vi "autoMaintainCurrentInstructions.vi"(6 "error in (no error)":errorcluster, 7 "MotionProfile acceleration":dbl[](array[numeric]), 8 "MotionProfile speed":dbl[](array[numeric]), 9 "running commands":string[][](array[string])) -> (0 "error out":errorcluster, 3 "running commands out":string[][](array[string]))   [LabVIEW 2012]
uses:
  <vilib>/addons/control/pid/pid.llb/PID (DBL).vi
  <vilib>/addons/control/pid/NI_PID_pid.lvlib
panel:
  in  "gyro PID":T1={"proportional gain (Kc)"=0.03, "integral time (Ti, min)"=0.01, "derivative time (Td, min)"=0.0} {"derivative time (Td, min)" format="%.3f"; "integral time (Ti, min)" format="%.3f"; "proportional gain (Kc)" format="%.3f"}
  in  "BasicDriveOffset 2":dbl=1.07
  in  "visionDrive output range":cluster{"output high":dbl, "output low":dbl}={"output high"=0.3, "output low"=-0.3} {"output low" format="%.2f"; "output high" format="%.2f"}
  in  "visionDrive PID":T1={"proportional gain (Kc)"=-2.5, "integral time (Ti, min)"=0.0, "derivative time (Td, min)"=0.0} {"derivative time (Td, min)" format="%.3f"; "integral time (Ti, min)" format="%.3f"; "proportional gain (Kc)" format="%.3f"}
  in  "manualDrivePID":T1={"proportional gain (Kc)"=1.0, "integral time (Ti, min)"=0.01, "derivative time (Td, min)"=0.0} {"derivative time (Td, min)" format="%.3f"; "integral time (Ti, min)" format="%.3f"; "proportional gain (Kc)" format="%.3f"}
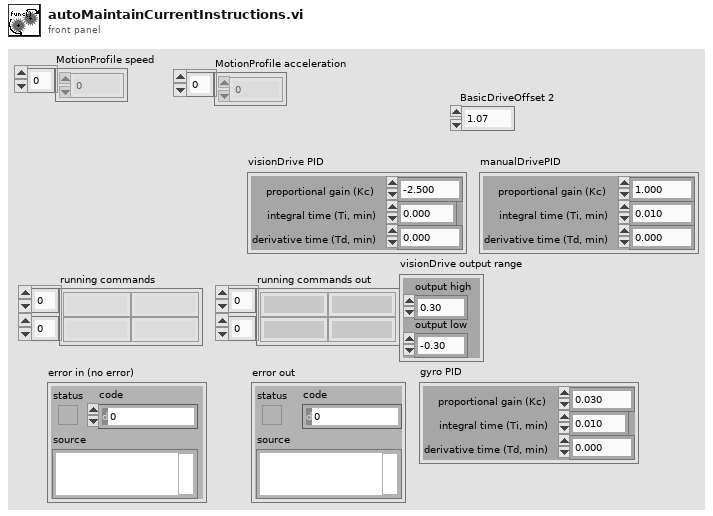
[diagram p1: front panel]
types:
  T1 = cluster{"proportional gain (Kc)":dbl, "integral time (Ti, min)":dbl, "derivative time (Td, min)":dbl}
  T2 = typedef "WPI_GyroDevRef.ctl" = cluster{"DevStatus":errorcluster, "Analog Module":T3, "Analog Channel":T4, "Offset":dbl, "Gain (VoltsPerDegree/Second)":dbl}
  T3 = typedef "FPGA_TypedefAnalogModule.ctl" = enum16{"Analog Module 1", "Analog Module 2"}
  T4 = typedef "FPGA_AIChannel.ctl" = enum8{"AI 1", "AI 2", "AI 3", "AI 4", "AI 5", "AI 6", "AI 7", "AI 8", "Invalid"}
  T5 = typedef "WPI_EncoderDevRef.ctl" = cluster{"DevStatus":errorcluster, "EncoderIndex":T6, "CounterIndex":T7, "DistancePerCount":dbl, "Decoding Type":T8}
  T6 = typedef "FPGA_EncoderIdx.ctl" = enum8{"Enc 0", "Enc 1", "Enc 2", "Enc 3", "Invalid"}
  T7 = typedef "FPGA_CounterCtrSystemIndex.ctl" = enum8{"Ctr 0", "Ctr 1", "Ctr 2", "Ctr 3", "Ctr 4", "Ctr 5", "Ctr 6", "Ctr 7", "Invalid"}
  T8 = typedef "WPI_EncoderType.ctl" = enum16{"1x", "2x", "4x"}
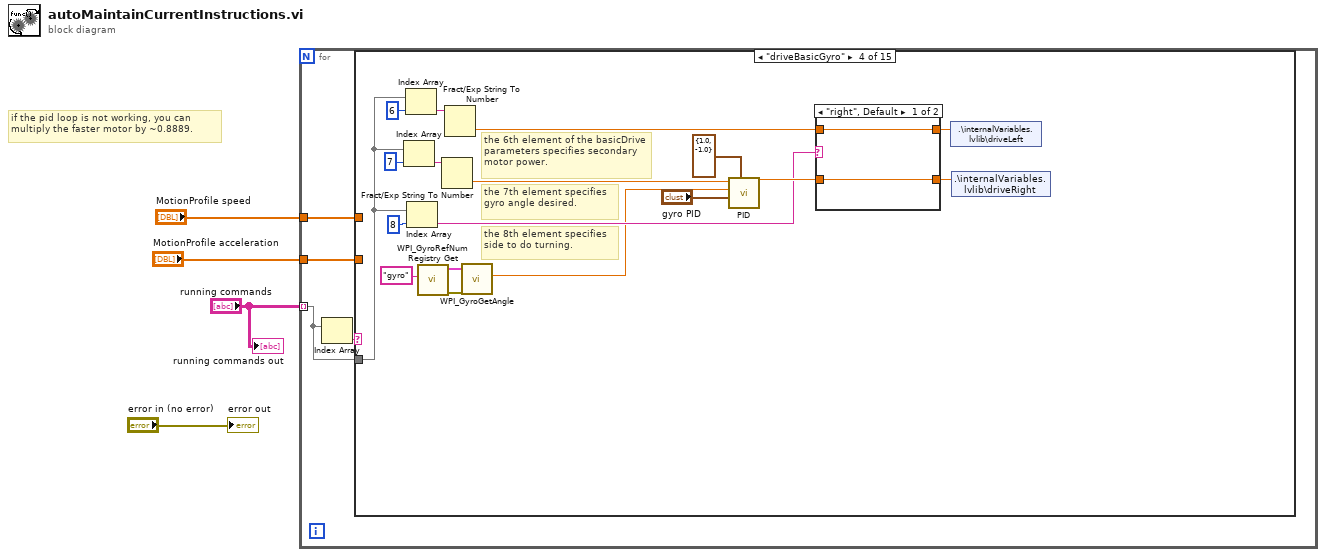
[diagram p0: block diagram]
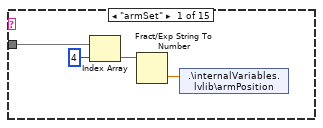
[diagram p2: hidden frame]
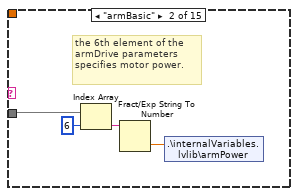
[diagram p3: hidden frame]
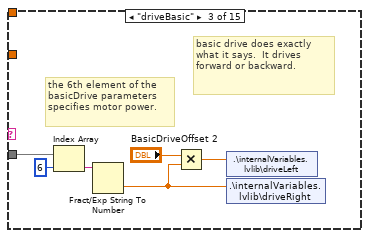
[diagram p4: hidden frame]
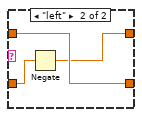
[diagram p5: hidden frame]
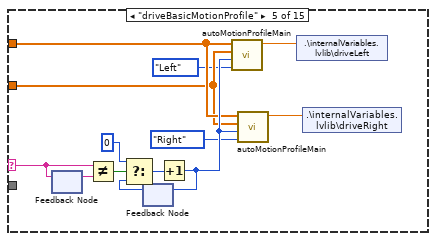
[diagram p6: hidden frame]
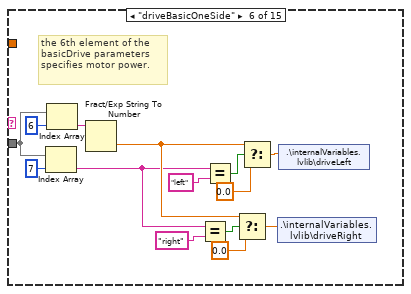
[diagram p7: hidden frame]
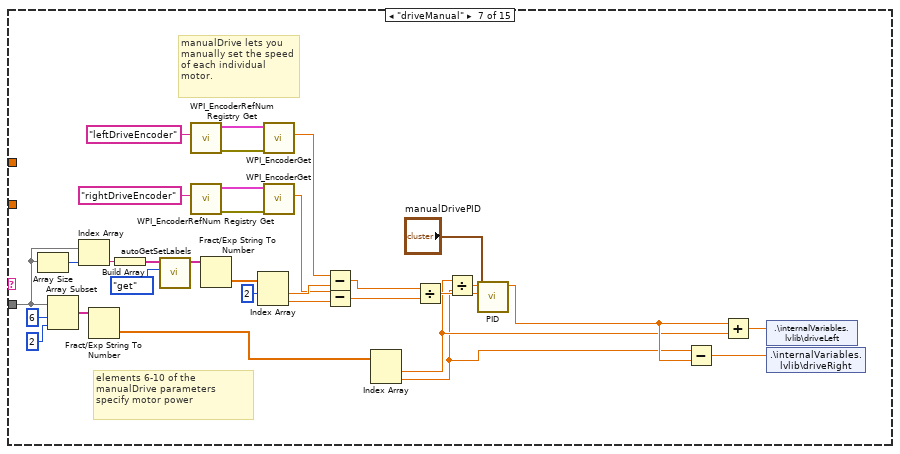
[diagram p8: hidden frame]
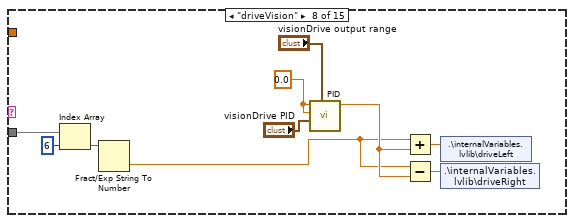
[diagram p9: hidden frame]
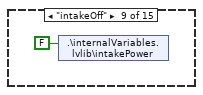
[diagram p10: hidden frame]
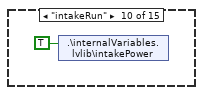
[diagram p11: hidden frame]
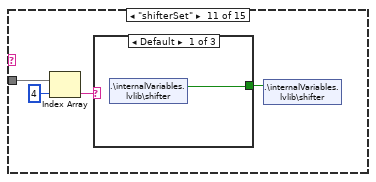
[diagram p12: hidden frame]
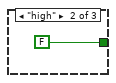
[diagram p13: hidden frame]
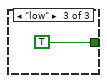
[diagram p14: hidden frame]
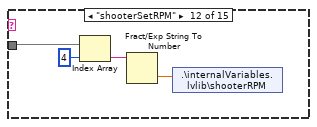
[diagram p15: hidden frame]
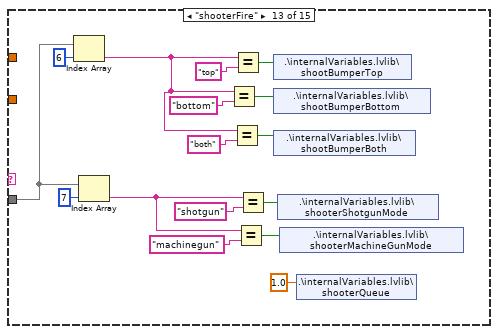
[diagram p16: hidden frame]
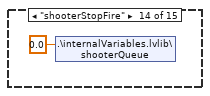
[diagram p17: hidden frame]
diagram:
  # "if the pid loop is not working, you can multiply the faster motor by ~0.8889."
  n1 = for {
    tunnel: "running commands" -> [w7] mode=indexing
    tunnel: "MotionProfile speed" -> [w6]
    tunnel: "MotionProfile acceleration" -> [w5]
    n2 = Index Array(array=w7) -> (element=w8:string)  [unwired: 1 in]
    n3 = case shown="\"driveBasicGyro\"" w8 {
      selector: w8 -> [_ _ _ _ w58 _ _ _ _ _ _ _ _ _ _]
      tunnel: w7 -> [w10 w13 w18 w34 _ w69 w96 w107 _ _ w120 w126 w134 _ _]
      tunnel: w6 -> [_ _ _ _ w49 _ _ _ _ _ _ _ _ _ _]
      tunnel: w5 -> [_ _ _ _ w48 _ _ _ _ _ _ _ _ _ _]
      frame "armSet" {
        n4 = Index Array(array=w10, index=4) -> (element=w12:string)
        n5 = Fract/Exp String To Number(string=w12) -> (number=w9:dbl)  [unwired: 3 in, 1 out]
        n6 = shared-variable ".\\internalVariables.lvlib\\armPosition"(w9) -> ()  [unwired: 1 in, 1 out]
      }
      frame "armBasic" {
        # "the 6th element of the armDrive parameters specifies motor power."
        n7 = Index Array(array=w13, index=6) -> (element=w15:string)
        n8 = Fract/Exp String To Number(string=w15) -> (number=w14:dbl)  [unwired: 3 in, 1 out]
        n9 = shared-variable ".\\internalVariables.lvlib\\armPower"(w14) -> ()  [unwired: 1 in, 1 out]
      }
      frame "driveBasic" {
        # "basic drive does exactly what it says.  It drives forward or backward."
        # "the 6th element of the basicDrive parameters specifies motor power."
        n10 = Index Array(array=w18, index=6) -> (element=w21:string)
        n11 = Fract/Exp String To Number(string=w21) -> (number=w17:dbl)  [unwired: 3 in, 1 out]
        n12 = Multiply(x="BasicDriveOffset 2", y=w17) -> (x*y=w20:dbl)
        n13 = shared-variable ".\\internalVariables.lvlib\\driveLeft"(w20) -> ()  [unwired: 1 in, 1 out]
        n14 = shared-variable ".\\internalVariables.lvlib\\driveRight"(w17) -> ()  [unwired: 1 in, 1 out]
      }
      frame "driveBasicGyro" {
        # "the 8th element specifies side to do turning."
        # "the 7th element specifies gyro angle desired."
        # "the 6th element of the basicDrive parameters specifies secondary motor power."
        n15 = Index Array(array=w34, index=7) -> (element=w35:string)
        n16 = Index Array(array=w34, index=6) -> (element=w39:string)
        n17 = Index Array(array=w34, index=8) -> (element=w28:string)
        n18 = call <vilib>:"WPI_GyroRefNum Registry Get.vi"("refnum name"="gyro") -> ("error out"=w26:errorcluster, "GyroDevRef"=w25:T2)  [unwired: 9 in]
        n19 = Fract/Exp String To Number(string=w35) -> (number=w27:dbl)  [unwired: 3 in, 1 out]
        n20 = Fract/Exp String To Number(string=w39) -> (number=w31:dbl)  [unwired: 3 in, 1 out]
        n21 = call <vilib>:"WPI_GyroGetAngle.vi"("error in (no error)"=w26, "GyroDevRef"=w25) -> ("Angle"=w24:dbl)  [unwired: 6 in, 3 out]
        n22 = call-poly <vilib>:"PID.vi"("output range"=cluster{"output high":dbl, "output low":dbl} {"output high"=1.0, "output low"=-1.0}, "PID gains"="gyro PID", "process variable"=w24, "setpoint"=w27) -> ("output"=w32:dbl)  [unwired: 6 in, 1 out]
        n23 = case shown="\"right\", Default" w28 {
          tunnel: w32 -> [w42 w44]
          tunnel: [w42 w45] -> w30
          tunnel: w31 -> [w41 w45]
          tunnel: [w41 w43] -> w29
          frame "right", Default {
          }
          frame "left" {
            n24 = Negate(x=w44) -> (-x=w43:dbl)
          }
        }
        n25 = shared-variable ".\\internalVariables.lvlib\\driveLeft"(w29) -> ()  [unwired: 1 in, 1 out]
        n26 = shared-variable ".\\internalVariables.lvlib\\driveRight"(w30) -> ()  [unwired: 1 in, 1 out]
      }
      frame "driveBasicMotionProfile" {
        n27 = feedback-in #1(w58) -> ()
        n28 = feedback #1() -> (w57:string)  [unwired: 1 in]
        n29 = Not Equal?(x=w58, y=w57) -> (x != y?=w56:bool)
        n30 = feedback #2() -> (w53:i32)  [unwired: 1 in]
        n31 = Select(t=0, s=w56, f=w53) -> (s? t:f=w54:i32)
        n32 = Increment(x=w54) -> (x+1=w50:i32)
        n33 = feedback-in #2(w50) -> ()
        n34 = call "autoMotionProfileMain.vi"("Drivetrain Side"=enum16{"Left", "Right"}."Left", "Counter"=w50, "Acceleration steps"=w48, "Speed steps"=w49) -> ("MotorPower"=w52:dbl)  [unwired: 7 in]
        n35 = call "autoMotionProfileMain.vi"("Drivetrain Side"=enum16{"Left", "Right"}."Right", "Counter"=w50, "Acceleration steps"=w48, "Speed steps"=w49) -> ("MotorPower"=w51:dbl)  [unwired: 7 in]
        n36 = shared-variable ".\\internalVariables.lvlib\\driveLeft"(w52) -> ()  [unwired: 1 in, 1 out]
        n37 = shared-variable ".\\internalVariables.lvlib\\driveRight"(w51) -> ()  [unwired: 1 in, 1 out]
      }
      frame "driveBasicOneSide" {
        # "the 6th element of the basicDrive parameters specifies motor power."
        n38 = Index Array(array=w69, index=7) -> (element=w60:string)
        n39 = Index Array(array=w69, index=6) -> (element=w72:string)
        n40 = Fract/Exp String To Number(string=w72) -> (number=w61:dbl)  [unwired: 3 in, 1 out]
        n41 = Equal?(x=w60, y="right") -> (x = y?=w59:bool)
        n42 = Equal?(x=w60, y="left") -> (x = y?=w67:bool)
        n43 = Select(t=w61, s=w59, f=0.0) -> (s? t:f=w62:dbl)
        n44 = Select(t=w61, s=w67, f=0.0) -> (s? t:f=w65:dbl)
        n45 = shared-variable ".\\internalVariables.lvlib\\driveRight"(w62) -> ()  [unwired: 1 in, 1 out]
        n46 = shared-variable ".\\internalVariables.lvlib\\driveLeft"(w65) -> ()  [unwired: 1 in, 1 out]
      }
      frame "driveManual" {
        # "manualDrive lets you manually set the speed of each individual motor."
        # "elements 6-10 of the manualDrive parameters specify motor power"
        n47 = Array Size(array=w96) -> (size(s)=w98:i32)
        n48 = Array Subset(array=w96, index=6, length=2) -> (w102:string[])
        n49 = Index Array(array=w96, index=w98) -> (element=w97:string)
        n50 = Fract/Exp String To Number(string=w102) -> (number=w101:dbl[])  [unwired: 3 in, 1 out]
        n51 = Build Array(w97) -> (w99:string[])
        n52 = call "autoGetSetLabels.vi"("option in"=enum16{"get", "set", "remove", "set end"}."get", "label in"=w99) -> ("label out"=w88:string[])  [unwired: 9 in]
        n53 = call <vilib>:"WPI_EncoderRefNum Registry Get.vi"("refnum name"="leftDriveEncoder") -> ("error out"=w94:errorcluster, "EncoderDevRef"=w95:T5)  [unwired: 9 in]
        n54 = call <vilib>:"WPI_EncoderRefNum Registry Get.vi"("refnum name"="rightDriveEncoder") -> ("error out"=w91:errorcluster, "EncoderDevRef"=w90:T5)  [unwired: 9 in]
        n55 = Fract/Exp String To Number(string=w88) -> (number=w87:dbl[])  [unwired: 3 in, 1 out]
        n56 = Index Array(array=w87, index #1=2 ("index")) -> (element #1=w85:dbl, element #2=w83:dbl)  [unwired: 1 in]
        n57 = call <vilib>:"WPI_EncoderGet.vi"("error in (no error)"=w94, "EncoderDevRef"=w95) -> ("Distance"=w86:dbl)  [unwired: 4 in, 5 out]
        n58 = call <vilib>:"WPI_EncoderGet.vi"("error in (no error)"=w91, "EncoderDevRef"=w90) -> ("Distance"=w84:dbl)  [unwired: 4 in, 5 out]
        n59 = Subtract(x=w86, y=w85) -> (x-y=w80:dbl)
        n60 = Subtract(x=w84, y=w83) -> (x-y=w79:dbl)
        n61 = Index Array(array=w101) -> (element #1=w75:dbl, element #2=w74:dbl)  [unwired: 2 in]
        n62 = Divide(x=w80, y=w79) -> (x/y=w82:dbl)
        n63 = Divide(x=w75, y=w74) -> (x/y=w81:dbl)
        n64 = call-poly <vilib>:"PID.vi"("PID gains"="manualDrivePID", "process variable"=w82, "setpoint"=w81) -> ("output"=w76:dbl)  [unwired: 7 in, 1 out]
        n65 = Subtract(x=w74, y=w76) -> (x-y=w73:dbl)
        n66 = Add(x=w76, y=w75) -> (x+y=w77:dbl)
        n67 = shared-variable ".\\internalVariables.lvlib\\driveLeft"(w77) -> ()  [unwired: 1 in, 1 out]
        n68 = shared-variable ".\\internalVariables.lvlib\\driveRight"(w73) -> ()  [unwired: 1 in, 1 out]
      }
      frame "driveVision" {
        w105 = 0.0 ("setpoint")
        n69 = Index Array(array=w107, index=6) -> (element=w113:string)
        n70 = Fract/Exp String To Number(string=w113) -> (number=w110:dbl)  [unwired: 3 in, 1 out]
        n71 = call-poly <vilib>:"PID.vi"("output range"="visionDrive output range", "PID gains"="visionDrive PID", "process variable"=w105, "setpoint"=w105) -> ("output"=w111:dbl)  [unwired: 6 in, 1 out]
        n72 = Add(x=w110, y=w111) -> (x+y=w109:dbl)
        n73 = Subtract(x=w110, y=w111) -> (x-y=w108:dbl)
        n74 = shared-variable ".\\internalVariables.lvlib\\driveLeft"(w109) -> ()  [unwired: 1 in, 1 out]
        n75 = shared-variable ".\\internalVariables.lvlib\\driveRight"(w108) -> ()  [unwired: 1 in, 1 out]
      }
      frame "intakeOff" {
        n76 = shared-variable ".\\internalVariables.lvlib\\intakePower"(FALSE ("intakePower")) -> ()  [unwired: 1 in, 1 out]
      }
      frame "intakeRun" {
        n77 = shared-variable ".\\internalVariables.lvlib\\intakePower"(TRUE ("intakePower")) -> ()  [unwired: 1 in, 1 out]
      }
      frame "shifterSet" {
        n78 = Index Array(array=w120, index=4) -> (element=w119:string)
        n79 = case shown="Default" w119 {
          tunnel: [w121 FALSE ("driveShifterLow") TRUE ("driveShifterLow")] -> w118
          frame Default {
            n80 = shared-variable ".\\internalVariables.lvlib\\shifter"() -> (w121:bool)  [unwired: 1 in, 1 out]
          }
          frame "high" {
          }
          frame "low" {
          }
        }
        n81 = shared-variable ".\\internalVariables.lvlib\\shifter"(w118) -> ()  [unwired: 1 in, 1 out]
      }
      frame "shooterSetRPM" {
        n82 = Index Array(array=w126, index=4) -> (element=w125:string)
        n83 = Fract/Exp String To Number(string=w125) -> (number=w124:dbl)  [unwired: 3 in, 1 out]
        n84 = shared-variable ".\\internalVariables.lvlib\\shooterRPM"(w124) -> ()  [unwired: 1 in, 1 out]
      }
      frame "shooterFire" {
        n85 = Index Array(array=w134, index=6) -> (element=w139:string)
        n86 = Index Array(array=w134, index=7) -> (element=w131:string)
        n87 = Equal?(x=w139, y="bottom") -> (x = y?=w137:bool)
        n88 = Equal?(x=w139, y="both") -> (x = y?=w138:bool)
        n89 = Equal?(x=w139, y="top") -> (x = y?=w136:bool)
        n90 = Equal?(x=w131, y="machinegun") -> (x = y?=w130:bool)
        n91 = Equal?(x=w131, y="shotgun") -> (x = y?=w129:bool)
        n92 = shared-variable ".\\internalVariables.lvlib\\shootBumperTop"(w136) -> ()  [unwired: 1 in, 1 out]
        n93 = shared-variable ".\\internalVariables.lvlib\\shootBumperBottom"(w137) -> ()  [unwired: 1 in, 1 out]
        n94 = shared-variable ".\\internalVariables.lvlib\\shootBumperBoth"(w138) -> ()  [unwired: 1 in, 1 out]
        n95 = shared-variable ".\\internalVariables.lvlib\\shooterShotgunMode"(w129) -> ()  [unwired: 1 in, 1 out]
        n96 = shared-variable ".\\internalVariables.lvlib\\shooterMachineGunMode"(w130) -> ()  [unwired: 1 in, 1 out]
        n97 = shared-variable ".\\internalVariables.lvlib\\shooterQueue"(1.0 ("shooterQueue")) -> ()  [unwired: 1 in, 1 out]
      }
      frame "shooterStopFire" {
        n98 = shared-variable ".\\internalVariables.lvlib\\shooterQueue"(0.0 ("shooterQueue")) -> ()  [unwired: 1 in, 1 out]
      }
      frame "testFunct", Default {
        # "This just acts as a time delay."
      }
    }
  }
  "running commands out" <- "running commands"
  "error out" <- "error in (no error)"
